vi "Get Mac Address.vi"(8 "error in (no error)":errorcluster, 10 "buffer":string, 11 "_hResourceContext":u32) -> (0 "error out":errorcluster, 2 "buffer out":string, 3 "_hResourceContext out":u32)   [LabVIEW 2013, in "QCAWLAN_DLL.lvlib"]
doc: "QCA_DLL_Export void GetMacAddress(HANDLE _hResourceContext, char *buffer);"
uses:
  QCAWLAN_DLL.lvlib
  QCAWLAN_DLL.dll
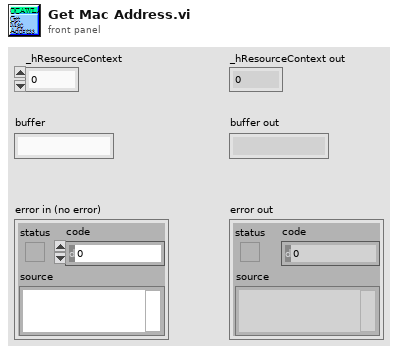
[diagram p1: front panel]
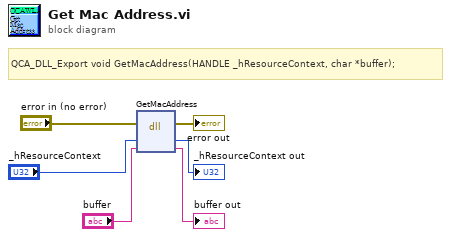
[diagram p0: block diagram]
diagram:
  # "QCA_DLL_Export void GetMacAddress(HANDLE _hResourceContext, char *buffer);"
  n1 = dll-call lib="C:/Connectivity Client - MIMO/PlugIn/QCAWLAN_DLL.*" fn="GetMacAddress"(error in="error in (no error)", "_hResourceContext"="_hResourceContext", "buffer"="buffer") -> (error out=→"error out":errorcluster, "_hResourceContext"=→"_hResourceContext out":u32, "buffer"=→"buffer out":string)  [unwired: 3 in, 1 out]
